vi "Copy target.vi"() -> ()   [LabVIEW 2014]
panel:
  in  "LabVIEW Class:Open":refnum<vi>
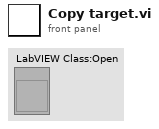
[diagram p1: front panel]
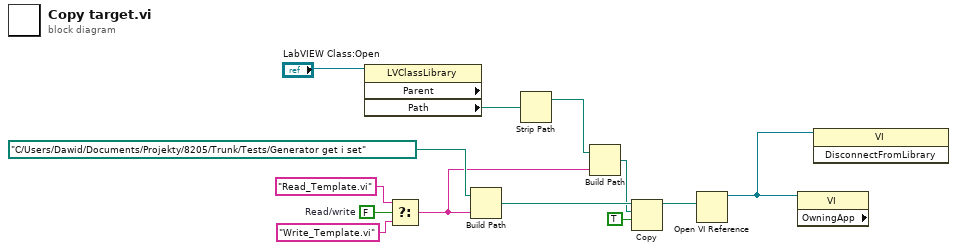
[diagram p0: block diagram]
diagram:
  w11 = FALSE  # Read/write
  n1 = property class="LVClassLibrary" props=["Parent", "Path"](reference="LabVIEW Class:Open") -> ("Path"=w12:path)  [unwired: 1 in, 3 out]
  n2 = Select(t="Read_Template.vi", s=w11, f="Write_Template.vi") -> (s? t:f=w4:string)
  n3 = Build Path(base path=path "C:/Users/Dawid/Documents/Projekty/8205/Trunk/Tests/Generator get i set" ("Path"), name or relative path=w4) -> (appended path=w7:path)
  n4 = Strip Path(path=w12) -> (stripped path=w5:path)  [unwired: 1 out]
  n5 = Build Path(base path=w5, name or relative path=w4) -> (appended path=w3:path)
  n6 = Copy(9:TRUE ("overwrite (F)"), 10:w3, 11:w7) -> (3:w2:path)  [unwired: 2 in, 2 out]
  n7 = Open VI Reference(vi path=w2) -> (vi reference=w1:refnum<vi>)  [unwired: 5 in, 1 out]
  n8 = property class="VI" props=["OwningApp"](reference=w1) -> ()  [unwired: 1 in, 3 out]
  n9 = invoke class="VI" method="DisconnectFromLibrary"(reference=w1) -> ()  [unwired: 2 in, 3 out]
